vi "OMV_Initialize.vi"(11 "VISA Refnum in":refnum<visa-resource-name>) -> (0 "error out":errorcluster, 3 "VISA Refnum out":refnum<visa-resource-name>)   [LabVIEW 2017]
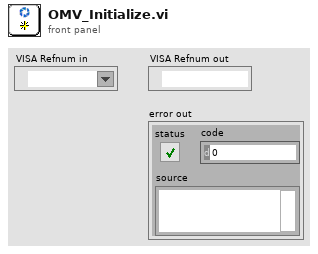
[diagram p1: front panel]
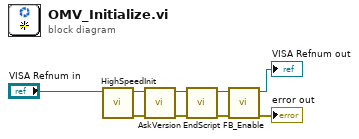
[diagram p0: block diagram]
diagram:
  n1 = call <userlib>:"HighSpeedInit.vi"("VISA Refnum in"="VISA Refnum in") -> ("error out"=w5:errorcluster, "VISA Refnum out"=w6:refnum<visa-resource-name>)  [unwired: 9 in]
  n2 = call <userlib>:"AskVersion.vi"("error in"=w5, "VISA Refnum in"=w6) -> ("error out"=w8:errorcluster, "VISA Refnum out"=w9:refnum<visa-resource-name>)  [unwired: 7 in, 1 out]
  n3 = call <userlib>:"EndScript.vi"("error in (no error)"=w8, "VISA Refnum in"=w9) -> ("error out"=w2:errorcluster, "VISA Refnum out"=w4:refnum<visa-resource-name>)  [unwired: 7 in, 1 out]
  n4 = call <userlib>:"FB_Enable.vi"("error in"=w2, "VISA Refnum in"=w4) -> ("error out"=→"error out":errorcluster, "VISA Refnum out"=→"VISA Refnum out":refnum<visa-resource-name>)  [unwired: 7 in, 1 out]
